vi "ROI grp-Save Load Groups header-Core.vi"(8 "error in (no error)":errorcluster, 9 "POI groups header file data (& header) to save":string[][](array[string]), 10 "Function":T1, 11 "Experiment folder path":path) -> (0 "error out":errorcluster, 2 "Loaded POI groups header":string[](array[string]), 3 "Loaded POI groups table data (No header)":string[][](array[string]))   [LabVIEW 2013]
uses:
  Experiment header interface/Typedefs/Save-Load-Save as-Load last enum.ctl
  Program Files (x86)/National Instruments/LabVIEW 2013/user.lib/My Palettes.lib/Files & paths/Spreadsheet/Write To Spreadsheet File (string)-Mod.vi
  Program Files (x86)/National Instruments/LabVIEW 2013/user.lib/My Palettes.lib/Files & paths/Spreadsheet/Read From Spreadsheet File (string)-Mod.vi
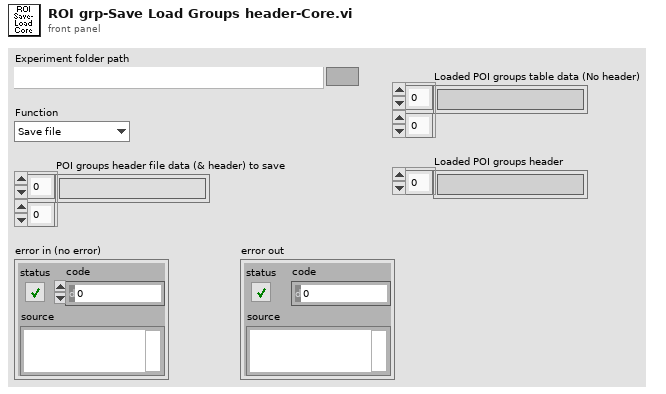
[diagram p1: front panel]
types:
  T1 = typedef "Save-Load-Save as-Load last enum.ctl" = enum16{"Save file", "Save file as", "Load file", "Load last file"}
  T2 = typedef "Fixed strings.ctl" = cluster{"ROI file name":string, "Normalised ROI file name":string, "Zplane Pockels values file name":string, "Functional data folder name":string, "Experiment Header file name":string, "Z-stack images folder name":string, "Groups setup rel. path":string, "Groups text file rel. path":string, "TDMS files folder name (F.img)":string, "TDMS files folder name (V.acq)":string, "TDMS files folder name (Pl.acq)":string, "Cycle rel times sequence file":string, "Dynamically called VIs folder name":string, "Time Series folder base name":string}
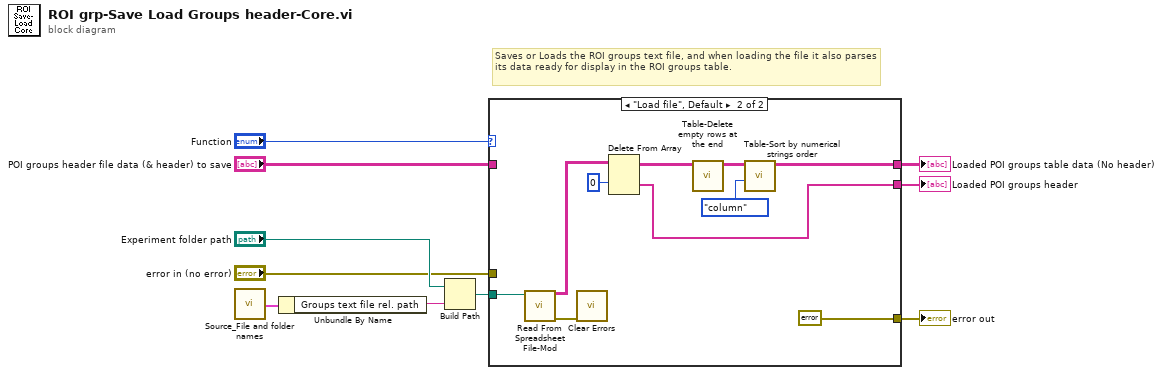
[diagram p0: block diagram]
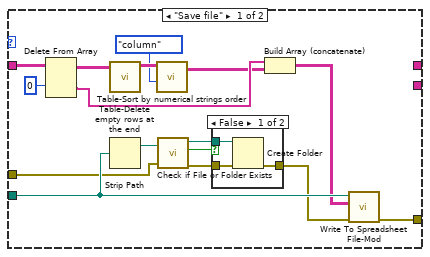
[diagram p2: hidden frame]
diagram:
  # "Saves or Loads the ROI groups text file, and when loading the file it also parses its data ready for display in the ROI groups table."
  n1 = call "Source_File and folder names.vi"() -> ("Fixed strings"=w1:T2)  [unwired: 1 in]
  n2 = Unbundle By Name(w1) -> ("Groups text file rel. path"=w2:string)
  n3 = Build Path(base path="Experiment folder path", name or relative path=w2) -> (appended path=w5:path)
  n4 = case shown="\"Load file\", Default" "Function" {
    tunnel: [w19 errorcluster {"status"=FALSE, "code"=0, "source"=""} ("error out")] -> w4
    tunnel: w5 -> [w24 w40]
    tunnel: "POI groups header file data (& header) to save" -> [w15 _]
    tunnel: [_ w32] -> w6
    tunnel: "error in (no error)" -> [w22 _]
    tunnel: [_ w31] -> w8
    frame "Save file" {
      n5 = Delete From Array(array=w15, index (row)=0) -> (deleted portion=w13:string[], array with subset deleted=w14:string[][])  [unwired: 2 in]
      n6 = call "Table-Delete empty rows at the end.vi"("Value in"=w14) -> ("Value out"=w18:string[][])  [unwired: 10 in]
      n7 = Strip Path(path=w24) -> (stripped path=w23:path)  [unwired: 1 out]
      n8 = call "Table-Sort by numerical strings order.vi"("Sort By in"=enum16{"row", "column"}."column", "Numerical strings table in"=w18) -> ("Sorted numerical strings table"=w12:string[][])  [unwired: 8 in, 1 out]
      n9 = call <vilib>:"Check if File or Folder Exists.vi"("error in (no error)"=w22, "path"=w23) -> ("error out"=w25:errorcluster, "file or folder exists?"=w21:bool, "dup path"=w26:path)  [unwired: 7 in]
      n10 = case shown="False" w21 {
        tunnel: w26 -> [w29 _]
        tunnel: w25 -> [w28 w30]
        tunnel: [w27 w30] -> w20
        frame False {
          n11 = Create Folder(path (use dialog)=w29, error in=w28) -> (error out=w27:errorcluster)  [unwired: 1 in, 2 out]
        }
        frame True {
        }
      }
      n12 = Build Array (concatenate)(w13, w12) -> (w11:string[][])
      n13 = call-poly "Write To Spreadsheet File-Mod.vi"("error in"=w20, "2D data"=w11, "file path (dialog if empty)"=w24) -> ("error out"=w19:errorcluster)  [unwired: 7 in, 1 out]
    }
    frame "Load file", Default {
      n14 = call-poly "Read From Spreadsheet File-Mod.vi"("file path (dialog if empty)"=w40) -> ("all rows"=w34:string[][], "error out"=w38:errorcluster)  [unwired: 9 in, 4 out]
      n15 = call <vilib>:"Clear Errors.vi"("error in (no error)"=w38) -> ()  [unwired: 6 in, 1 out]
      n16 = Delete From Array(array=w34, index (row)=0) -> (deleted portion=w31:string[], array with subset deleted=w33:string[][])  [unwired: 2 in]
      n17 = call "Table-Delete empty rows at the end.vi"("Value in"=w33) -> ("Value out"=w36:string[][])  [unwired: 10 in]
      n18 = call "Table-Sort by numerical strings order.vi"("Sort By in"=enum16{"row", "column"}."column", "Numerical strings table in"=w36) -> ("Sorted numerical strings table"=w32:string[][])  [unwired: 8 in, 1 out]
    }
  }
  "Loaded POI groups header" <- w8
  "Loaded POI groups table data (No header)" <- w6
  "error out" <- w4
